vi "BuildBattleSQLString.vi"(11 "BattleLog":T1) -> (3 "SQL INSERT request":string)   [LabVIEW 2020, in "StashRoyale.lvclass"]
uses:
  StashRoyale.lvclass
  ctl_BattleLog.ctl
  ctl_Team.ctl
  ctl_CardTeam.ctl
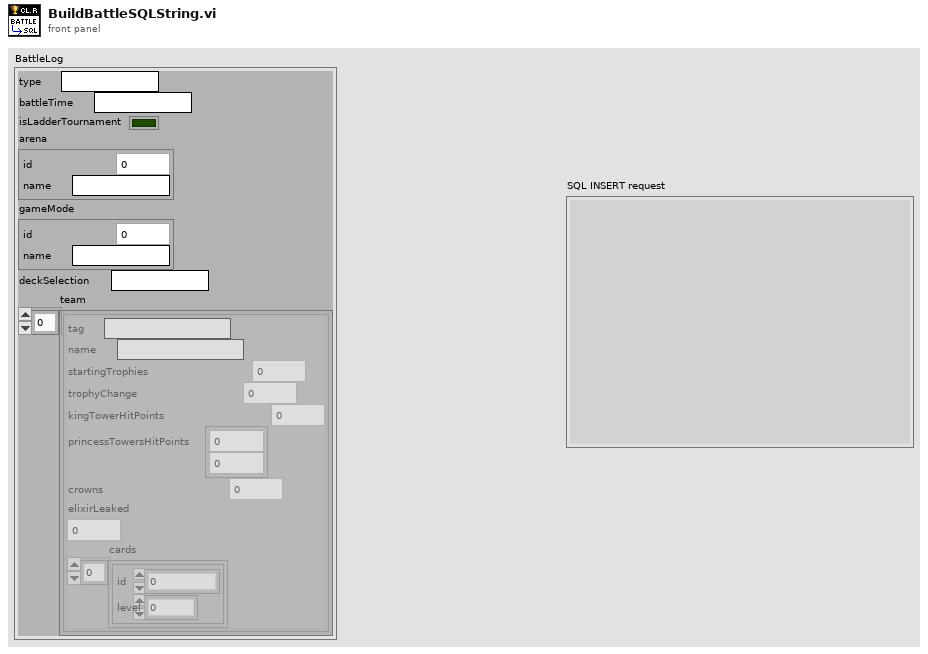
[diagram p1: front panel]
types:
  T1 = typedef "StashRoyale.lvclass/ctl_BattleLog.ctl" = cluster{"type":string, "battleTime":string, "isLadderTournament":bool, "arena":cluster{"id":u32, "name":string}, "gameMode":cluster{"id":u32, "name":string}, "deckSelection":string, "team":T2[]}
  T2 = typedef "ctl_Team.ctl" = cluster{"tag":string, "name":string, "startingTrophies":u16, "trophyChange":i16, "kingTowerHitPoints":u16, "princessTowersHitPoints":u16[], "crowns":u16, "elixirLeaked":sgl, "cards":T3[]}
  T3 = typedef "StashRoyale.lvclass/ctl_CardTeam.ctl" = cluster{"id":u32, "level":u8}
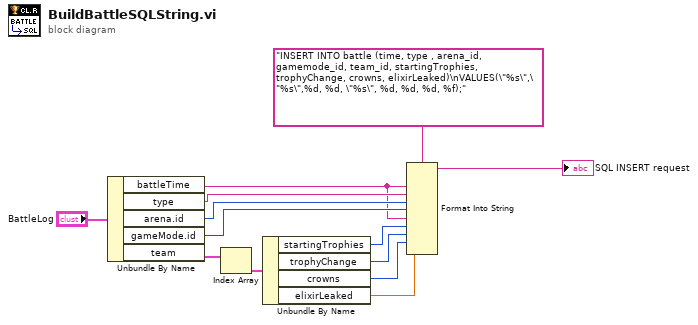
[diagram p0: block diagram]
diagram:
  n1 = Unbundle By Name("BattleLog") -> ("battleTime"=w5:string, "type"=w11:string, "arena.id"=w10:u32, "gameMode.id"=w9:u32, "team"=w8:T2[])
  n2 = Index Array(array=w8) -> (element=w7:T2)  [unwired: 1 in]
  n3 = Unbundle By Name(w7) -> ("startingTrophies"=w4:u16, "trophyChange"=w3:i16, "crowns"=w2:u16, "elixirLeaked"=w1:sgl)
  n4 = Format Into String(format string="INSERT INTO battle (time, type , arena_id, gamemode_id, team_id, startingTrophies, trophyChange, crowns, elixirLeaked)\nVALUES(\"%s\",\"%s\",%d, %d, \"%s\", %d, %d, %d, %f);", w5, w11, w10, w9, w5, w4, w3, w2, w1) -> (resulting string=→"SQL INSERT request":string)  [unwired: 2 in, 1 out]
